vi "Generator-facade.vi"(0 "Data In":T7={"Data"=0.0, "+"=FALSE, "-"=FALSE, "Output"=FALSE, "Power "=FALSE, "Ecran Power"="", "Ekran data"=0.0, "Coarse"=3.0, "Fine"=3.0}, 2 "Display State In":T5, 3 "Container State":T6) -> (6 "Data Out":T7={"Data"=0.0, "+"=FALSE, "-"=FALSE, "Output"=FALSE, "Power "=FALSE, "Ecran Power"="", "Ekran data"=0.0, "Coarse"=3.0, "Fine"=3.0}, 7 "Display State Out":T5, 8 "Action":T4)   [LabVIEW 2020, in "Generator.xctl"]
uses:
  Generator.xctl
  Generator-data.ctl
  Power Ecran.ctl
  Ecran data.ctl
  <vilib>/_xctls/Container State.ctl
  Generator-state.ctl
  <vilib>/_xctls/Action.ctl
  Coarse.ctl
  Fine.ctl
  <vilib>/_xctls/XControlSupport.lvlib
panel:
  out "Ekran data":T1
  in  "Fine [x100mV]":T2 scale=0.0..30.0
  in  "Coarse [V]":T3 scale=0.0..30.0
  in  "Power":bool
  in  "Output":bool
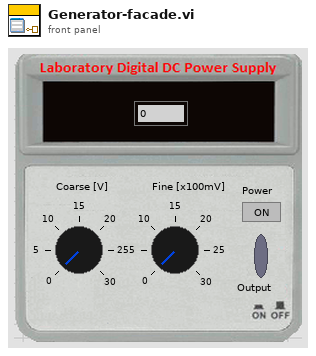
[diagram p1: front panel]
types:
  T1 = typedef "Ecran data.ctl" = dbl
  T2 = typedef "Fine.ctl" = dbl
  T3 = typedef "Coarse.ctl" = dbl
  T4 = typedef "XControlSupport.lvlib/Action.ctl" = cluster{"Data Changed?":bool, "State Changed?":bool, "Action Name":string}
  T5 = typedef "Generator.xctl/Generator-state.ctl" = cluster{"ON":bool, "Output":bool, "Connected?":bool}
  T6 = typedef "XControlSupport.lvlib/Container State.ctl" = cluster{"Indicator?":bool, "Run Mode?":bool, " Refnum":refnum<vi>}
  T7 = typedef "Generator.xctl/Generator-data.ctl" = cluster{"Data":dbl, "+":bool, "-":bool, "Output":bool, "Power ":bool, "Ecran Power":T8, "Ekran data":T1, "Coarse":dbl, "Fine":dbl}
  T8 = typedef "Power Ecran.ctl" = string
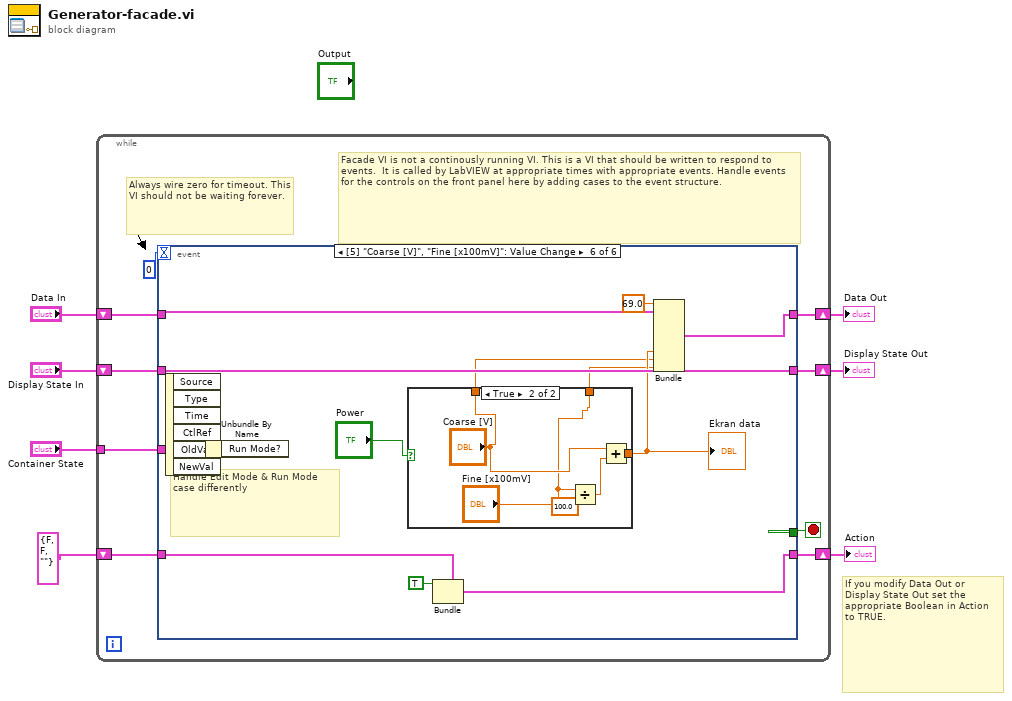
[diagram p0: block diagram]
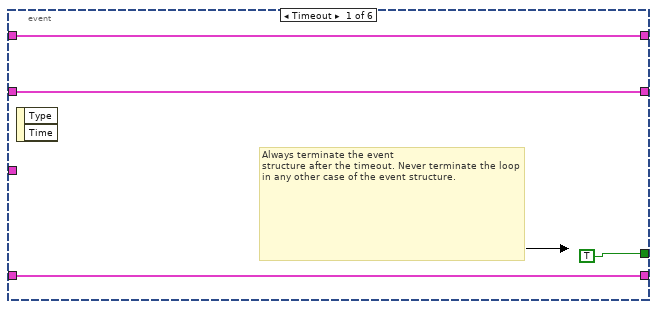
[diagram p2: hidden frame]
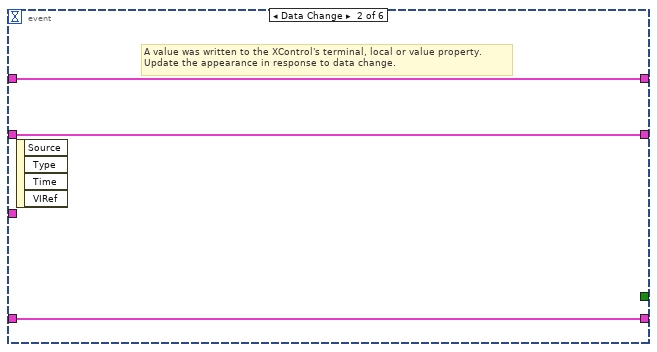
[diagram p3: hidden frame]
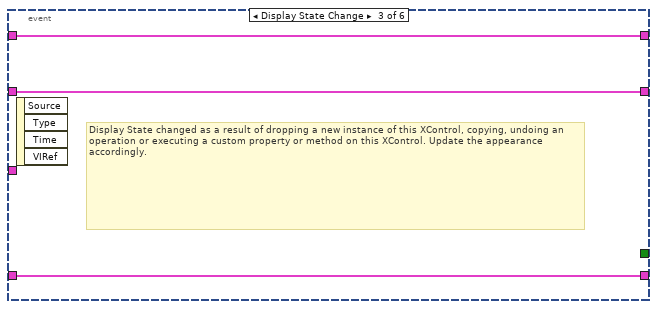
[diagram p4: hidden frame]
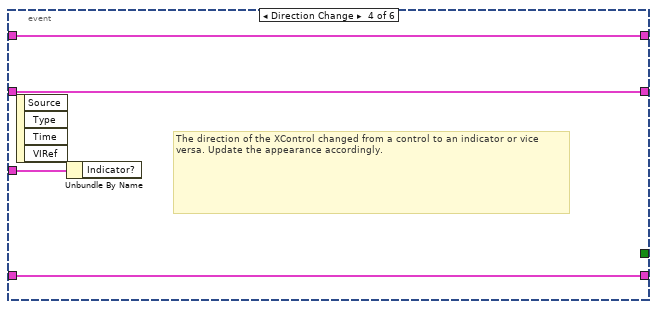
[diagram p5: hidden frame]
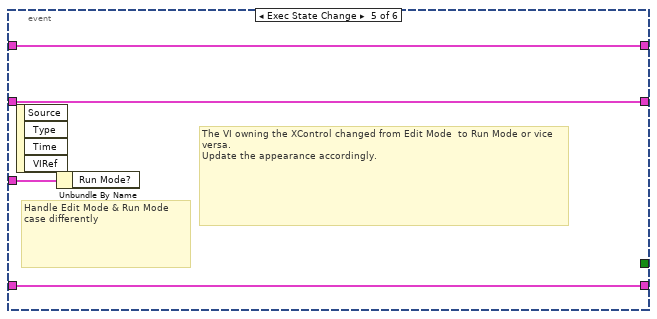
[diagram p6: hidden frame]
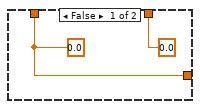
[diagram p7: hidden frame]
diagram:
  # "If you modify Data Out or\nDisplay State Out set the\nappropriate Boolean in Action\nto TRUE."
  n1 = while {
    shift-right: [w15] -> w4
    shift-left: "Display State In" -> [w16]
    tunnel: "Container State" -> [w12]
    shift-right: [w10] -> w7
    shift-left: "Data In" -> [w11]
    shift-right: [w8] -> w2
    shift-left: T4 {"Data Changed?"=FALSE, "State Changed?"=FALSE, "Action Name"=""} ("Action") -> [w9]
    stop <- w14 stop-if-true
    # "Facade VI is not a continously running VI. This is a VI that should be written to respond to events.  It is called by LabVIEW at appropriate times with appropriate events. Handle events for the controls on the front panel here by adding cases to the event structure."
    # "Always wire zero for timeout. This\nVI should not be waiting forever."
    n2 = event shown="[5] \"Coarse [V]\", \"Fine [x100mV]\": Value Change" {
      selector: _ -> [_ _ _ _ _ _]
      dyn-events: _ -> [_ _ _ _ _ _]
      timeout: 0 -> [_ _ _ _ _ _]
      tunnel: w16 -> [w18 w22 w26 w29 w33 w45]
      tunnel: [w18 w22 w26 w29 w33 w45] -> w15
      tunnel: [TRUE _ _ _ _ _] -> w14
      tunnel: w12 -> [_ _ _ w30 w34 w46]
      tunnel: w11 -> [w17 w21 w25 w28 w32 w44]
      tunnel: [w17 w21 w25 w28 w32 w43] -> w10
      tunnel: [w19 w23 w24 w27 w31 w36] -> w8
      tunnel: w9 -> [w19 w23 w24 w27 w31 w37]
      event Timeout {
        # "Always terminate the event\nstructure after the timeout. Never terminate the loop in any other case of the event structure."
        n3 = event-data() -> ()  [unwired: 1 in, 2 out]
      }
      event Data Change {
        # "A value was written to the XControl's terminal, local or value property.\nUpdate the appearance in response to data change."
        n4 = event-data() -> ()  [unwired: 1 in, 4 out]
      }
      event Display State Change {
        # "Display State changed as a result of dropping a new instance of this XControl, copying, undoing an operation or executing a custom property or method on this XControl. Update the appearance accordingly."
        n5 = event-data() -> ()  [unwired: 1 in, 4 out]
      }
      event Direction Change {
        # "The direction of the XControl changed from a control to an indicator or vice versa. Update the appearance accordingly."
        n6 = event-data() -> ()  [unwired: 1 in, 4 out]
        n7 = Unbundle By Name(w30) -> ()  [unwired: 1 out]
      }
      event Exec State Change {
        # "The VI owning the XControl changed from Edit Mode  to Run Mode or vice versa.\nUpdate the appearance accordingly."
        # "Handle Edit Mode & Run Mode\ncase differently"
        n8 = event-data() -> ()  [unwired: 1 in, 4 out]
        n9 = Unbundle By Name(w34) -> ()  [unwired: 1 out]
      }
      event Value Change {
        # "Handle Edit Mode & Run Mode\ncase differently"
        n10 = event-data() -> ()  [unwired: 1 in, 6 out]
        n11 = Unbundle By Name(w46) -> ()  [unwired: 1 out]
        n12 = case shown="True" "Power" {
          tunnel: [T2 0.0 ("Fine [x100mV]") "Fine [x100mV]"] -> w39
          tunnel: [w47 w52] -> w41
          tunnel: [w47 "Coarse [V]"] -> w40
          frame False {
            w47 = T3 0.0 ("Coarse [V]")
          }
          frame True {
            n13 = Divide(x="Fine [x100mV]", y=T2 100.0) -> (x/y=w51:T2)
            n14 = Add(x="Coarse [V]", y=w51) -> (x+y=w52:T3)
          }
        }
        "Ekran data" <- w41
        n15 = Bundle(cluster=w37, "Data Changed?"=TRUE) -> (w36:T4)  [unwired: 2 in]
        n16 = Bundle(cluster=w44, "Data"=69.0, "Ekran data"=w41, "Coarse"=w40, "Fine"=w39) -> (w43:T7)  [unwired: 5 in]
      }
    }
  }
  "Display State Out" <- w4
  "Data Out" <- w7
  "Action" <- w2
